vi "Feedback_Read (SubVI).vi"(5 "System State Feedback":i8[](array[numeric])=[90, -91, 10, -86, 1, 0, 0, 0, 0, 0, 0] format="%x") -> (2 "System Feedback code":u8[](array[numeric]), 3 "System Feedback":T5, 4 "Motion Feedback":T4, 6 "Motor 1 Feedback":T3, 8 "Motor 2 Feedback":T3, 10 "Motor 3 Feedback":T3, 14 "Light Feedback":T2, 15 "Motor 4 Feedback":T3)   [LabVIEW 2019]
uses:
  Ctrl/agv_status.ctl
panel:
  out "Motor feedback":T1
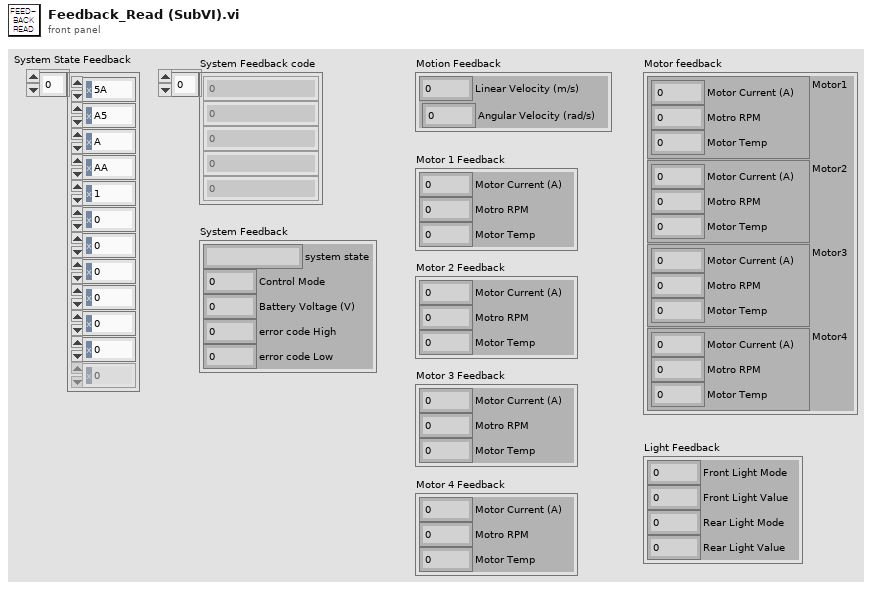
[diagram p1: front panel]
types:
  T1 = cluster{"Motor1":cluster{"Motor Current (A)":dbl, "Motro RPM":u16, "Motor Temp":i8}, "Motor2":cluster{"Motor Current (A)":dbl, "Motro RPM":u16, "Motor Temp":i8}, "Motor3":cluster{"Motor Current (A)":dbl, "Motro RPM":u16, "Motor Temp":i8}, "Motor4":cluster{"Motor Current (A)":dbl, "Motro RPM":u16, "Motor Temp":i8}}
  T2 = cluster{"Front Light Mode":i8, "Front Light Value":i8, "Rear Light Mode":i8, "Rear Light Value":i8}
  T3 = cluster{"Motor Current (A)":dbl, "Motro RPM":u16, "Motor Temp":i8}
  T4 = cluster{"Linear Velocity (m/s)":dbl, "Angular Velocity (rad/s)":dbl}
  T5 = cluster{"system state":string, "Control Mode":u8, "Battery Voltage (V)":dbl, "error code High":u8, "error code Low":u8}
  T6 = typedef "agv_status.ctl" = enum16{"system status in", "motor status in", "light status in", "read"}
  T7 = cluster{cluster{"system state":string, "Control Mode":u8, "Battery Voltage (V)":dbl, "error code High":u8, "error code Low":u8}, cluster{"Linear Velocity (m/s)":dbl, "Angular Velocity (rad/s)":dbl}}
  T8 = cluster{cluster{"Motor Current (A)":dbl, "Motro RPM":u16, "Motor Temp":i8}, cluster{"Motor Current (A)":dbl, "Motro RPM":u16, "Motor Temp":i8}, cluster{"Motor Current (A)":dbl, "Motro RPM":u16, "Motor Temp":i8}, cluster{"Motor Current (A)":dbl, "Motro RPM":u16, "Motor Temp":i8}}
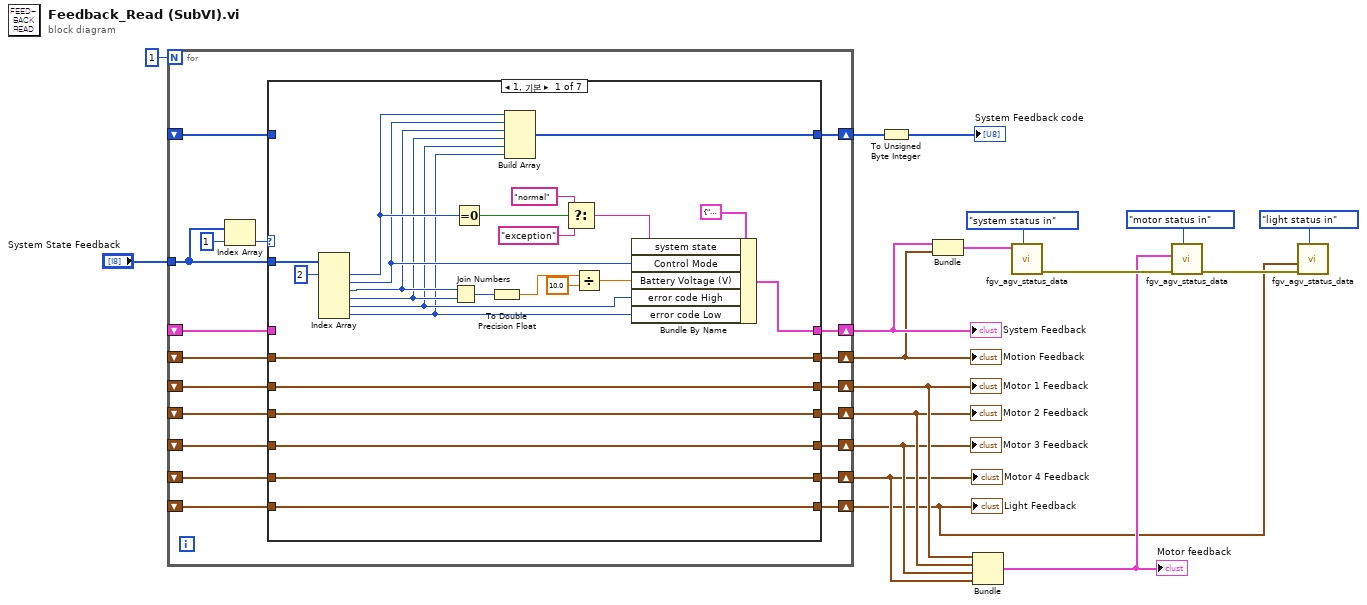
[diagram p0: block diagram]
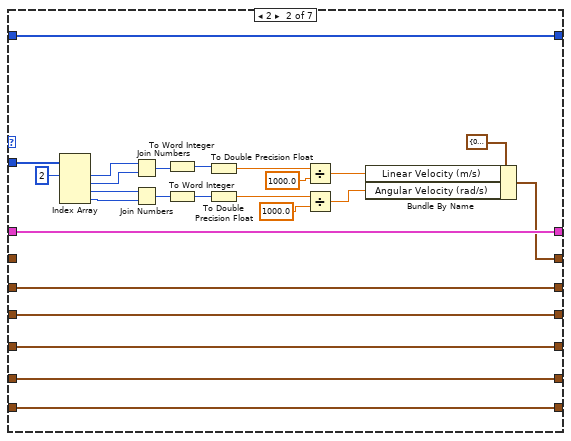
[diagram p2: hidden frame]
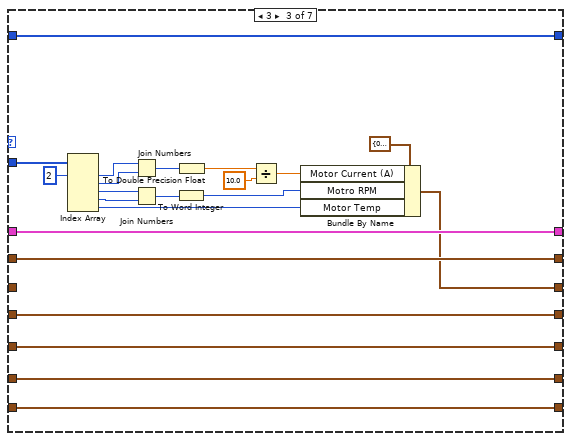
[diagram p3: hidden frame]
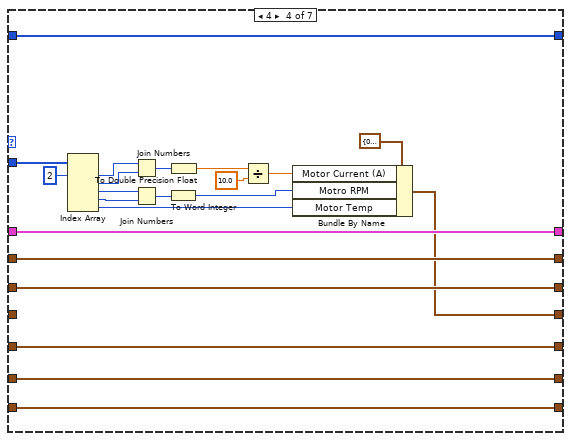
[diagram p4: hidden frame]
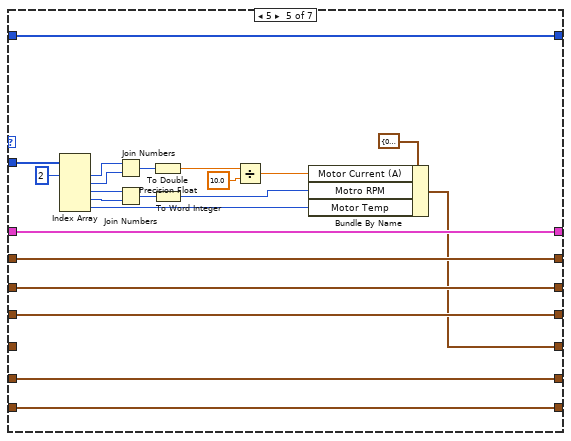
[diagram p5: hidden frame]
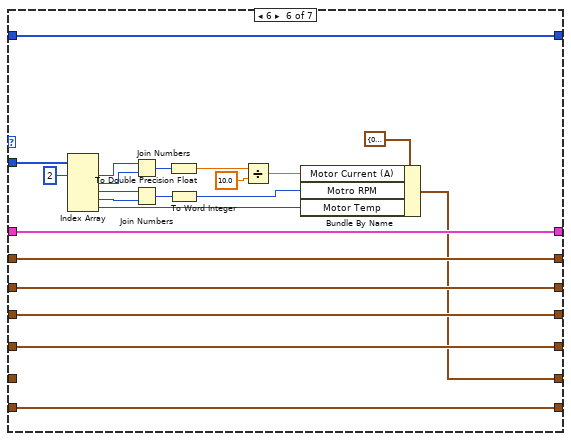
[diagram p6: hidden frame]
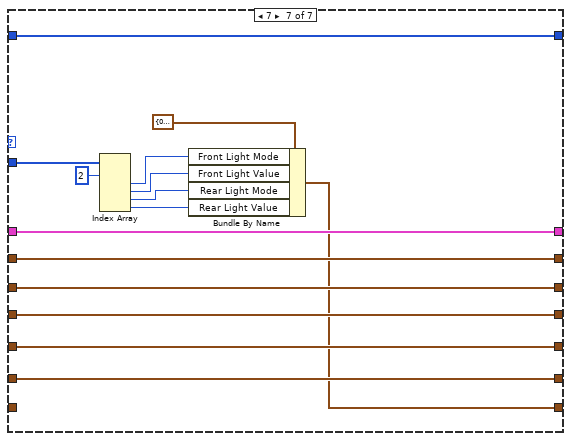
[diagram p7: hidden frame]
diagram:
  n1 = for {
    N: 1 -> [_]
    shift-right: [w34] -> w9
    shift-left: _ -> [w33]
    tunnel: "System State Feedback" -> [w35]
    shift-right: [w31] -> w8
    shift-left: _ -> [w32]
    shift-right: [w29] -> w14
    shift-left: _ -> [w30]
    shift-right: [w28] -> w13
    shift-left: _ -> [w27]
    shift-right: [w26] -> w12
    shift-left: _ -> [w25]
    shift-right: [w24] -> w11
    shift-left: _ -> [w23]
    shift-right: [w22] -> w3
    shift-left: _ -> [w21]
    shift-right: [w20] -> w17
    shift-left: _ -> [w19]
    n2 = Index Array(array=w35, index=1) -> (element=w36:i8)
    n3 = case shown="1, 기본" w36 {
      tunnel: w35 -> [w52 w80 w101 w120 w142 w164 w184]
      tunnel: [w51 w76 w97 w119 w141 w163 w183] -> w34
      tunnel: w33 -> [_ w76 w97 w119 w141 w163 w183]
      tunnel: w32 -> [w50 _ w96 w118 w140 w162 w182]
      tunnel: [w50 w75 w96 w118 w140 w162 w182] -> w31
      tunnel: w30 -> [w49 w74 _ w117 w139 w161 w181]
      tunnel: [w49 w74 w95 w117 w139 w161 w181] -> w29
      tunnel: [w48 w73 w94 w116 w138 w160 w180] -> w28
      tunnel: w27 -> [w48 w73 w94 _ w138 w160 w180]
      tunnel: [w47 w72 w93 w115 w137 w159 w179] -> w26
      tunnel: w25 -> [w47 w72 w93 w115 _ w159 w179]
      tunnel: [w46 w71 w92 w114 w136 w158 w178] -> w24
      tunnel: w23 -> [w46 w71 w92 w114 w136 _ w178]
      tunnel: [w45 w70 w91 w113 w135 w157 w177] -> w22
      tunnel: w21 -> [w45 w70 w91 w113 w135 w157 _]
      tunnel: [w38 w63 w88 w110 w132 w154 w176] -> w20
      tunnel: w19 -> [_ w63 w88 w110 w132 w154 w176]
      frame 1, Default {
        n4 = Index Array(array=w52, index #1=2 ("index")) -> (element #1=w44:i8, element #2=w43:i8, element #3=w42:i8, element #4=w41:i8, element #5=w40:i8, element #6=w39:i8)  [unwired: 5 in]
        n5 = Join Numbers(hi=w42, lo=w41) -> ((hi.lo)=w59:u16)
        n6 = Equal To 0?(x=w44) -> (x = 0?=w58:bool)
        n7 = To Double Precision Float(number=w59) -> (double precision float=w60:dbl)
        n8 = Build Array(w44, w43, w42, w41, w40, w39) -> (w38:i8[])
        n9 = Select(t="normal", s=w58, f="exception") -> (s? t:f=w61:string)
        n10 = Divide(x=w60, y=10.0) -> (x/y=w62:dbl)
        n11 = Bundle By Name(cluster=T5 {"system state"="", "Control Mode"=0, "Battery Voltage (V)"=0.0, "error code High"=0, "error code Low"=0}, "system state"=w61, "Control Mode"=w43, "Battery Voltage (V)"=w62, "error code High"=w40, "error code Low"=w39) -> (w51:T5)
      }
      frame 2 {
        n12 = Index Array(array=w80, index #1=2 ("index")) -> (element #1=w69:i8, element #2=w68:i8, element #3=w86:i8, element #4=w85:i8)  [unwired: 3 in]
        n13 = Join Numbers(hi=w69, lo=w68) -> ((hi.lo)=w67:u16)
        n14 = Join Numbers(hi=w86, lo=w85) -> ((hi.lo)=w64:u16)
        n15 = To Word Integer(number=w67) -> (16bit integer=w66:i16)
        n16 = To Word Integer(number=w64) -> (16bit integer=w65:i16)
        n17 = To Double Precision Float(number=w66) -> (double precision float=w82:dbl)
        n18 = To Double Precision Float(number=w65) -> (double precision float=w84:dbl)
        n19 = Divide(x=w82, y=1000.0) -> (x/y=w78:dbl)
        n20 = Divide(x=w84, y=1000.0) -> (x/y=w77:dbl)
        n21 = Bundle By Name(cluster=T4 {"Linear Velocity (m/s)"=0.0, "Angular Velocity (rad/s)"=0.0}, "Linear Velocity (m/s)"=w78, "Angular Velocity (rad/s)"=w77) -> (w75:T4)
      }
      frame 3 {
        n22 = Index Array(array=w101, index #1=2 ("index")) -> (element #1=w103:i8, element #2=w102:i8, element #3=w108:i8, element #4=w107:i8, element #5=w98:i8)  [unwired: 4 in]
        n23 = Join Numbers(hi=w103, lo=w102) -> ((hi.lo)=w106:u16)
        n24 = Join Numbers(hi=w108, lo=w107) -> ((hi.lo)=w89:u16)
        n25 = To Word Integer(number=w89) -> (16bit integer=w90:i16)
        n26 = To Double Precision Float(number=w106) -> (double precision float=w105:dbl)
        n27 = Divide(x=w105, y=10.0) -> (x/y=w99:dbl)
        n28 = Bundle By Name(cluster=T3 {"Motor Current (A)"=0.0, "Motro RPM"=0, "Motor Temp"=0}, "Motor Current (A)"=w99, "Motro RPM"=w90, "Motor Temp"=w98) -> (w95:T3)
      }
      frame 4 {
        n29 = Index Array(array=w120, index #1=2 ("index")) -> (element #1=w128:i8, element #2=w129:i8, element #3=w124:i8, element #4=w125:i8, element #5=w131:i8)  [unwired: 4 in]
        n30 = Join Numbers(hi=w128, lo=w129) -> ((hi.lo)=w126:u16)
        n31 = Join Numbers(hi=w124, lo=w125) -> ((hi.lo)=w112:u16)
        n32 = To Word Integer(number=w112) -> (16bit integer=w111:i16)
        n33 = To Double Precision Float(number=w126) -> (double precision float=w127:dbl)
        n34 = Divide(x=w127, y=10.0) -> (x/y=w130:dbl)
        n35 = Bundle By Name(cluster=T3 {"Motor Current (A)"=0.0, "Motro RPM"=0, "Motor Temp"=0}, "Motor Current (A)"=w130, "Motro RPM"=w111, "Motor Temp"=w131) -> (w116:T3)
      }
      frame 5 {
        n36 = Index Array(array=w142, index #1=2 ("index")) -> (element #1=w147:i8, element #2=w146:i8, element #3=w152:i8, element #4=w151:i8, element #5=w143:i8)  [unwired: 4 in]
        n37 = Join Numbers(hi=w147, lo=w146) -> ((hi.lo)=w150:u16)
        n38 = Join Numbers(hi=w152, lo=w151) -> ((hi.lo)=w134:u16)
        n39 = To Double Precision Float(number=w150) -> (double precision float=w149:dbl)
        n40 = To Word Integer(number=w134) -> (16bit integer=w133:i16)
        n41 = Divide(x=w149, y=10.0) -> (x/y=w144:dbl)
        n42 = Bundle By Name(cluster=T3 {"Motor Current (A)"=0.0, "Motro RPM"=0, "Motor Temp"=0}, "Motor Current (A)"=w144, "Motro RPM"=w133, "Motor Temp"=w143) -> (w137:T3)
      }
      frame 6 {
        n43 = Index Array(array=w164, index #1=2 ("index")) -> (element #1=w169:i8, element #2=w168:i8, element #3=w174:i8, element #4=w173:i8, element #5=w165:i8)  [unwired: 4 in]
        n44 = Join Numbers(hi=w169, lo=w168) -> ((hi.lo)=w172:u16)
        n45 = Join Numbers(hi=w174, lo=w173) -> ((hi.lo)=w156:u16)
        n46 = To Double Precision Float(number=w172) -> (double precision float=w171:dbl)
        n47 = To Word Integer(number=w156) -> (16bit integer=w155:i16)
        n48 = Divide(x=w171, y=10.0) -> (x/y=w166:dbl)
        n49 = Bundle By Name(cluster=T3 {"Motor Current (A)"=0.0, "Motro RPM"=0, "Motor Temp"=0}, "Motor Current (A)"=w166, "Motro RPM"=w155, "Motor Temp"=w165) -> (w158:T3)
      }
      frame 7 {
        n50 = Index Array(array=w184, index #1=2 ("index")) -> (element #2=w188:i8, element #3=w187:i8, element #4=w186:i8, element #5=w185:i8)  [unwired: 4 in, 1 out]
        n51 = Bundle By Name(cluster=T2 {"Front Light Mode"=0, "Front Light Value"=0, "Rear Light Mode"=0, "Rear Light Value"=0}, "Front Light Mode"=w188, "Front Light Value"=w187, "Rear Light Mode"=w186, "Rear Light Value"=w185) -> (w177:T2)
      }
    }
  }
  "System Feedback" <- w9
  "Motion Feedback" <- w8
  "Motor 1 Feedback" <- w14
  "Motor 2 Feedback" <- w13
  "Motor 3 Feedback" <- w12
  "Motor 4 Feedback" <- w11
  "Light Feedback" <- w3
  n52 = To Unsigned Byte Integer(number=w17) -> (unsigned 8bit integer=→"System Feedback code":u8[])
  n53 = Bundle(w9, w8) -> (w7:T7)  [unwired: 1 in]
  n54 = Bundle(w14, w13, w12, w11) -> (w4:T8)  [unwired: 1 in]
  "Motor feedback" <- w4
  n55 = call "fgv_agv_status_data.vi"("cmd"=agv_status."system status in", "AGV status in"=w7) -> ("error out"=w6:errorcluster)  [unwired: 6 in, 3 out]
  n56 = call "fgv_agv_status_data.vi"("cmd"=agv_status."motor status in", "error in"=w6, "Motor status in"=w4) -> ("error out"=w5:errorcluster)  [unwired: 5 in, 3 out]
  n57 = call "fgv_agv_status_data.vi"("cmd"=agv_status."light status in", "error in"=w5, "Light status in"=w3) -> ()  [unwired: 5 in, 4 out]
